vi "Log Data.vi"   [LabVIEW 2014]
uses:
  <vilib>/Utility/config.llb/NI_LVConfig.lvlib
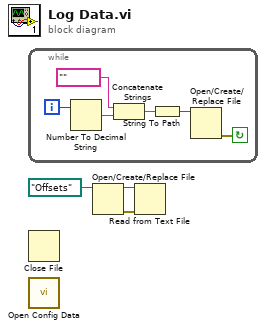
[diagram p0: block diagram]
diagram:
  n1 = while {
    i -> [w6]
    stop <- w9 continue-if-true
    n2 = Number To Decimal String(number=w6) -> (decimal integer string=w5:string)  [unwired: 1 in]
    n3 = Concatenate Strings("", w5) -> (w4:string)
    n4 = String To Path(string=w4) -> (path=w8:path)
    n5 = Open/Create/Replace File(file path (use dialog)=w8) -> (error out=w9:errorcluster)  [unwired: 5 in, 2 out]
  }
  n6 = Close File() -> ()  [unwired: 2 in, 2 out]
  n7 = call <vilib>:"Open Config Data.vi"() -> ()  [unwired: 9 in, 3 out]
  n8 = Open/Create/Replace File(file path (use dialog)=path "Offsets") -> (refnum out=w2:refnum<file>, error out=w1:errorcluster)  [unwired: 5 in, 1 out]
  n9 = Read from Text File(file (use dialog)=w2, error in=w1) -> ()  [unwired: 2 in, 4 out]
